vi "ni579x Construct Command Configure Clock.vi"(0 "Register Bus":refnum<class "ni579x Register Bus v1 Host.lvclass">=refnum, 1 "scope":string, 5 "clock source":string(combo), 7 "reference clock source":string(combo), 11 "Error In":errorcluster) -> (4 "Register Bus (out)":refnum<class "ni579x Register Bus v1 Host.lvclass">, 6 "User Command":T1 {"User Command ID" items=["Set Clock Select"=0, "Set CLK OUT Source"=1, "DAC Sync User Start"=2, "DAC Sync User End"=3, "Enable Baseband Amp"=5, "Set Rx Attenuation Pre-LNA"=7, "Set Rx Attenuation Post-LNA"=8, "Set Tx Attenuation"=9, "Set LO Filter"=32, "Set Front End Filter"=33, "Enable LO"=34, "Set Routing Mux"=37, "Read Current Rev Lower"=240, "Read Current Rev Upper"=241, "Read Oldest Compat Rev Lower"=242, "Read Oldest Compat Rev Upper"=243, "Re-Initialize"=255]; "User Data 1" format="%x"; "User Data 0" format="%x"}, 15 "Error Out":errorcluster)   [LabVIEW 2015]
uses:
  <instrlib>/ni579x/Register Bus/v1/Host/ni579x Register Bus v1 Host.lvclass
  <instrlib>/ni579x/Config/v1/Shared/Types/ni579x User Command.ctl
  <instrlib>/ni579x/Config/v1/Shared/Types/ni579x User Command ID.ctl
  <instrlib>/ni579x/Config/v1/Shared/Types/ni579x Clock Configuration.ctl
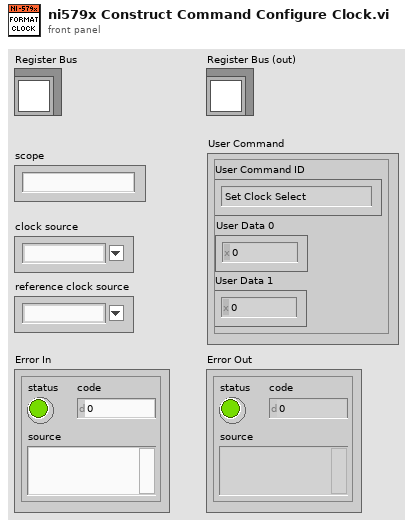
[diagram p1: front panel]
types:
  T1 = typedef "ni579x User Command.ctl" = cluster{"User Data 0":u8, "User Data 1":u8, "User Command ID":T2}
  T2 = typedef "ni579x User Command ID.ctl" = u8
  T3 = typedef "ni579x Clock Configuration.ctl" = u8
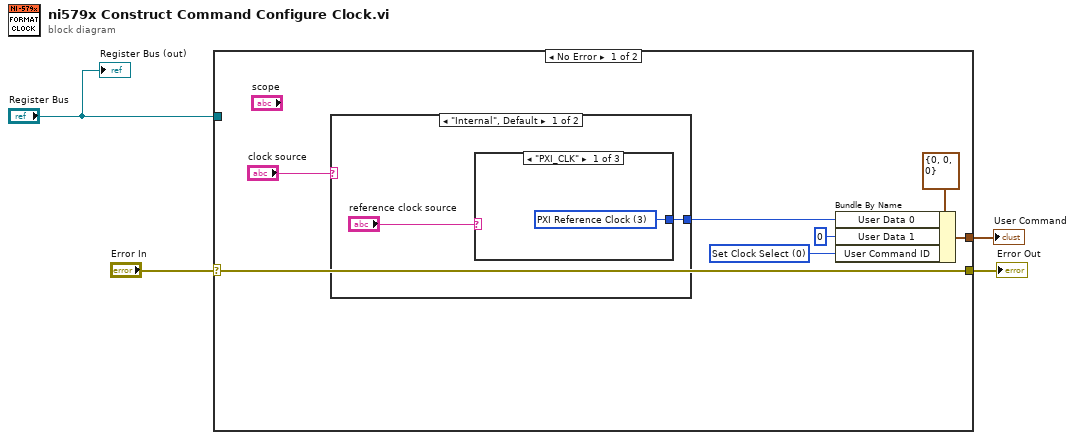
[diagram p0: block diagram]
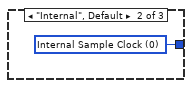
[diagram p2: hidden frame]
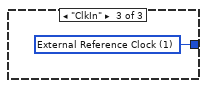
[diagram p3: hidden frame]
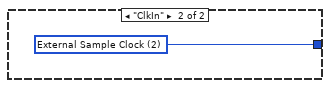
[diagram p4: hidden frame]
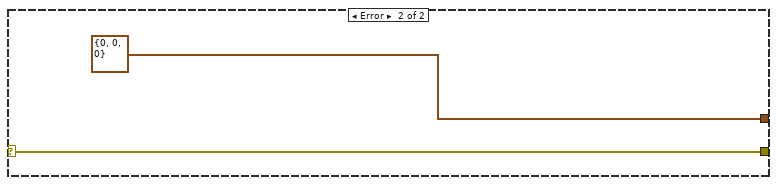
[diagram p5: hidden frame]
diagram:
  n1 = case shown="No Error" "Error In" {
    selector: "Error In" -> [w6 w19]
    tunnel: [w6 w19] -> w3
    tunnel: "Register Bus" -> [_ _]
    tunnel: [w10 T1 {"User Data 0"=0, "User Data 1"=0, "User Command ID"=0} ("User Command")] -> w1
    frame No Error {
      w5 = T2 0 items=["Set Clock Select"=0, "Set CLK OUT Source"=1, "DAC Sync User Start"=2, "DAC Sync User End"=3, "Enable Baseband Amp"=5, "Set Rx Attenuation Pre-LNA"=7, "Set Rx Attenuation Post-LNA"=8, "Set Tx Attenuation"=9, "Set LO Filter"=32, "Set Front End Filter"=33, "Enable LO"=34, "Set Routing Mux"=37, "Read Current Rev Lower"=240, "Read Current Rev Upper"=241, "Read Oldest Compat Rev Lower"=242, "Read Oldest Compat Rev Upper"=243, "Re-Initialize"=255] ("User Command ID")
      n2 = case shown="\"Internal\", Default" "clock source" {
        tunnel: [w12 w17] -> w7
        frame "Internal", Default {
          n3 = case shown="\"PXI_CLK\"" "reference clock source" {
            tunnel: [w14 w15 w16] -> w12
            frame "PXI_CLK" {
              w14 = T3 3 items=["Internal Sample Clock", "External Reference Clock", "External Sample Clock", "PXI Reference Clock"] ("Clock Configuration")
            }
            frame "Internal", Default {
              w15 = T3 0 items=["Internal Sample Clock", "External Reference Clock", "External Sample Clock", "PXI Reference Clock"] ("Clock Configuration")
            }
            frame "ClkIn" {
              w16 = T3 1 items=["Internal Sample Clock", "External Reference Clock", "External Sample Clock", "PXI Reference Clock"] ("Clock Configuration")
            }
          }
        }
        frame "ClkIn" {
          w17 = T3 2 items=["Internal Sample Clock", "External Reference Clock", "External Sample Clock", "PXI Reference Clock"] ("Clock Configuration")
        }
      }
      n4 = Bundle By Name(cluster=T1 {"User Data 0"=0, "User Data 1"=0, "User Command ID"=0} ("User Command"), "User Data 0"=w7, "User Data 1"=u8 0, "User Command ID"=w5) -> (w10:T1)
    }
    frame Error {
    }
  }
  "Error Out" <- w3
  "User Command" <- w1
  "Register Bus (out)" <- "Register Bus"
